vi "Register2.vi"(4 "Icp":i32(slide)=15 scale=0.0..15.0, 5 "Power Down":bool, 6 "Double Buff":bool, 7 "REF Divide":i16=1, 8 "REF /2":bool, 9 "REF X2":bool, 10 "MUX out":u16(ring)=4 items=["3-State", "GND", "Vcc", "Analog LD", "Digital LD", "REF / R", "RF / N"], 11 "Low Noise":bool=TRUE) -> (0 "HEX2":u32 format="%08x", 1 "Reg 2":bool[](array[boolean]))   [LabVIEW 2013]
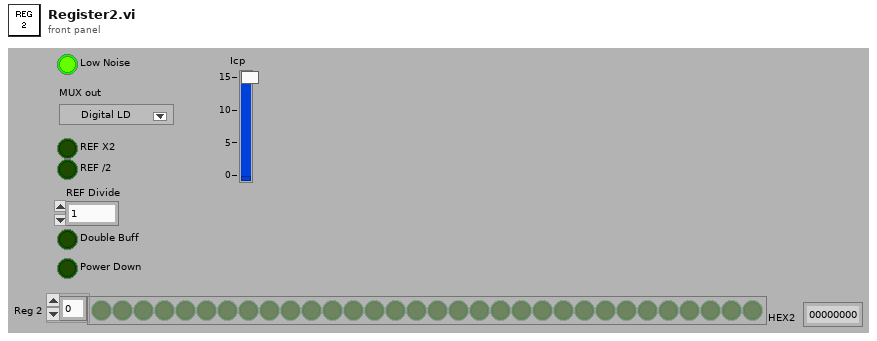
[diagram p1: front panel]
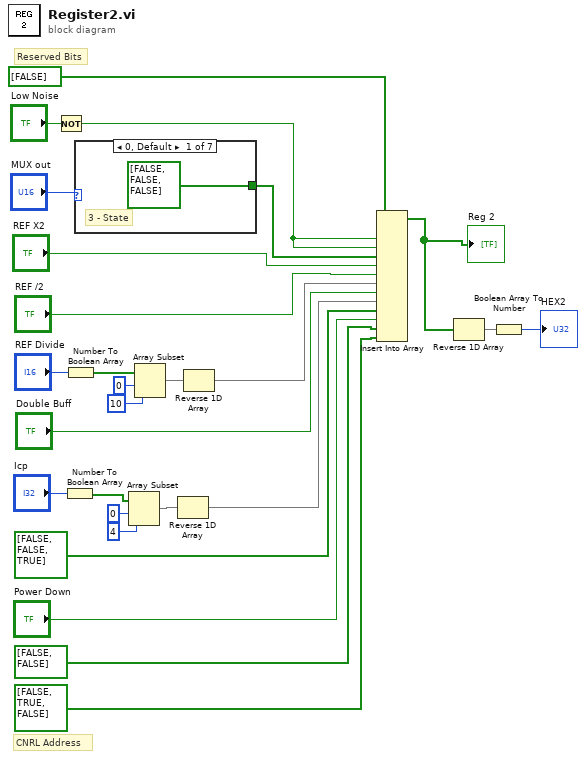
[diagram p0: block diagram]
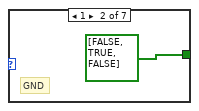
[diagram p2: hidden frame]
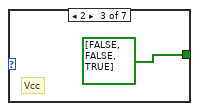
[diagram p3: hidden frame]
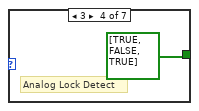
[diagram p4: hidden frame]
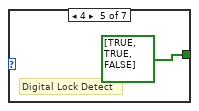
[diagram p5: hidden frame]
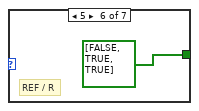
[diagram p6: hidden frame]
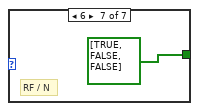
[diagram p7: hidden frame]
diagram:
  # "Reserved Bits"
  # "CNRL Address"
  n1 = Not(x="Low Noise") -> (.not. x?=w12:bool)
  n2 = Number To Boolean Array(number="Icp") -> (Boolean array=w25:bool[])
  n3 = Number To Boolean Array(number="REF Divide") -> (Boolean array=w18:bool[])
  n4 = case shown="0, Default" "MUX out" {
    tunnel: [bool[] [FALSE, FALSE, FALSE] bool[] [FALSE, TRUE, FALSE] bool[] [FALSE, FALSE, TRUE] bool[] [TRUE, FALSE, TRUE] bool[] [TRUE, TRUE, FALSE] bool[] [FALSE, TRUE, TRUE] bool[] [TRUE, FALSE, FALSE]] -> w10
    frame 0, Default {
      # "3 - State"
    }
    frame 1 {
      # "GND"
    }
    frame 2 {
      # "Vcc"
    }
    frame 3 {
      # "Analog Lock Detect"
    }
    frame 4 {
      # "Digital Lock Detect"
    }
    frame 5 {
      # "REF / R"
    }
    frame 6 {
      # "RF / N"
    }
  }
  n5 = Array Subset(array=w25, index=0, length=4) -> (w24:bool[])
  n6 = Array Subset(array=w18, index=0, length=10) -> (w17:bool[])
  n7 = Reverse 1D Array(array=w24) -> (reversed array=w5:bool[])
  n8 = Reverse 1D Array(array=w17) -> (reversed array=w7:bool[])
  n9 = Insert Into Array(array=bool[] [FALSE], new element #1=w12, new element #2=w12, new element #3=w10, new element #4="REF X2", new element #5="REF /2", new element #6=w7, new element #7="Double Buff", new element #8=w5, new element #9=bool[] [FALSE, FALSE, TRUE], new element #10="Power Down", new element #11=bool[] [FALSE, FALSE], new element #12=bool[] [FALSE, TRUE, FALSE]) -> (w14:bool[])  [unwired: 1 in]
  "Reg 2" <- w14
  n10 = Reverse 1D Array(array=w14) -> (reversed array=w21:bool[])
  n11 = Boolean Array To Number(Boolean array=w21) -> (number=→"HEX2":u32)
